vi "HexToString.vi"(11 "数组输入":u16[](array[numeric])) -> (3 "数组输出":string[](array[string]))   [LabVIEW 2016, in "超标留样集成.lvlib" / "ESTD1200.lvlib"]
uses:
  ESTD1200.lvlib
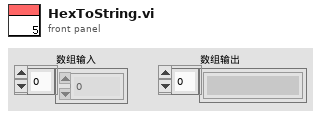
[diagram p1: front panel]
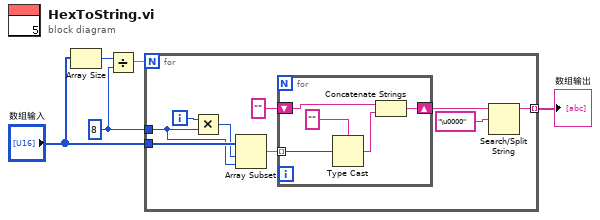
[diagram p0: block diagram]
diagram:
  w1 = 8 ("字符个数")
  n1 = Array Size(array="数组输入") -> (size(s)=w3:i32)
  n2 = Divide(x=w3, y=w1) -> (x/y=w2:dbl)
  n3 = for {
    N: w2 -> [_]
    tunnel: "数组输入" -> [w14]
    tunnel: [w8] -> w5 mode=indexing
    tunnel: w1 -> [w7]
    i -> [w13]
    n4 = Multiply(x=w13, y=w7) -> (x*y=w12:i32)
    n5 = Array Subset(array=w14, index=w12, length=w7) -> (w10:u16[])
    n6 = for {
      shift-right: [w19] -> w9
      shift-left: "" -> [w16]
      tunnel: w10 -> [w18] mode=indexing
      n7 = Type Cast(type="", x=w18) -> (*(type *) &x=w15:string)
      n8 = Concatenate Strings(w16, w15) -> (w19:string)
    }
    n9 = Search/Split String(string=w9, search string/char (-)="\u0000" ("搜索字符串")) -> (substring before match=w8:string)  [unwired: 1 in, 2 out]
  }
  "数组输出" <- w5
